vi "string test.vi"(11 "Array":string[][](array[string])) -> (2 "Modified Array Out":dbl[](array[numeric])=[2.0], 3 "Location":i32[][](array[numeric]))   [LabVIEW 2012]
uses:
  <vilib>/regexp/Match Regular Expression.xnode
panel:
  out "x >= 0?":bool
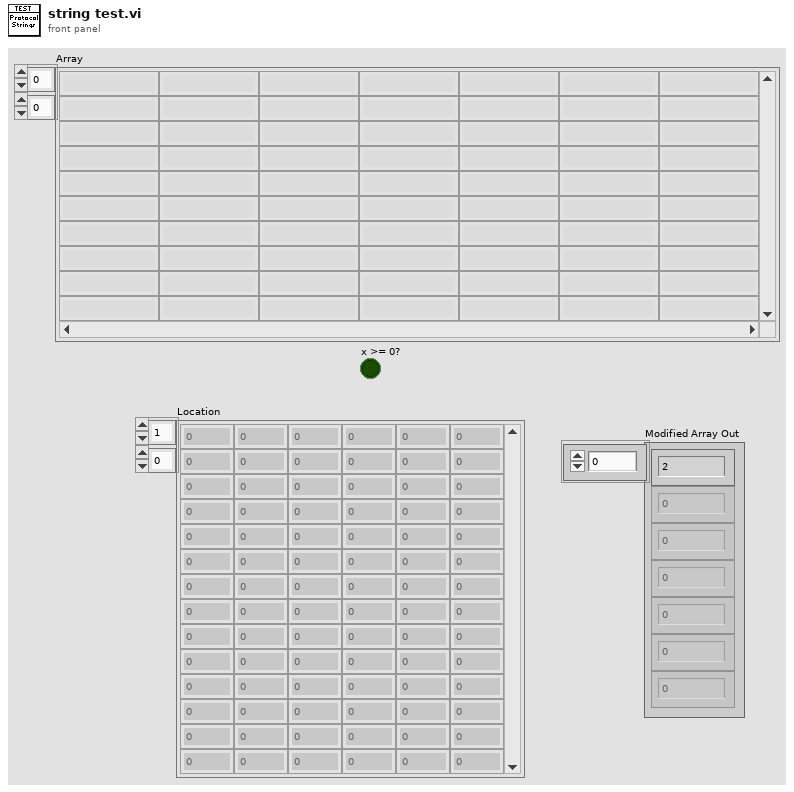
[diagram p1: front panel]
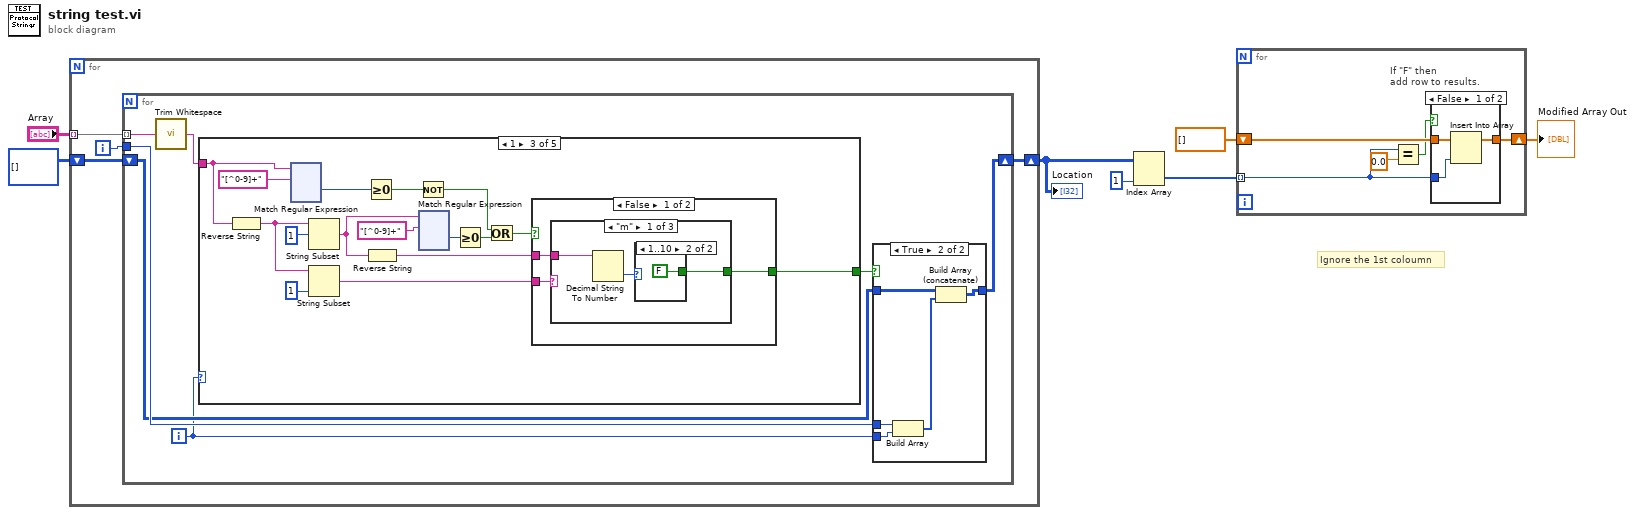
[diagram p0: block diagram]
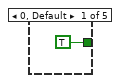
[diagram p4: hidden frame]
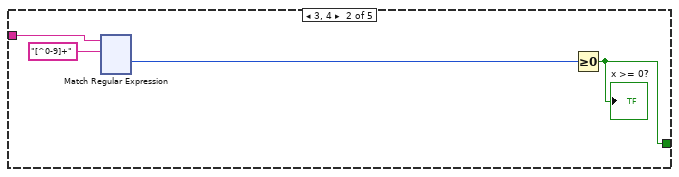
[diagram p5: hidden frame]
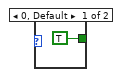
[diagram p6: hidden frame]
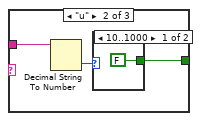
[diagram p7: hidden frame]
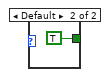
[diagram p8: hidden frame]
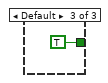
[diagram p9: hidden frame]
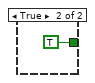
[diagram p10: hidden frame]
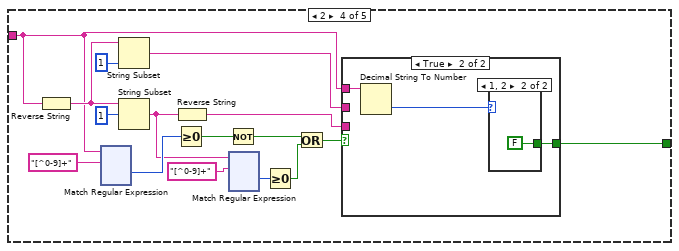
[diagram p11: hidden frame]
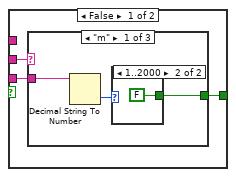
[diagram p12: hidden frame]
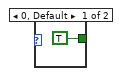
[diagram p13: hidden frame]
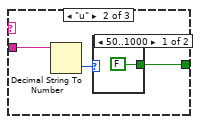
[diagram p14: hidden frame]
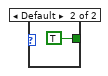
[diagram p15: hidden frame]
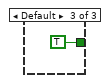
[diagram p16: hidden frame]
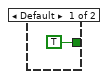
[diagram p17: hidden frame]
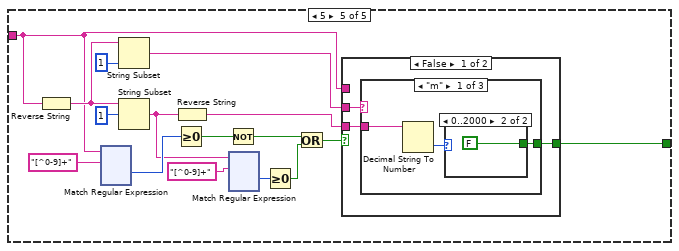
[diagram p18: hidden frame]
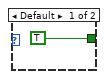
[diagram p19: hidden frame]
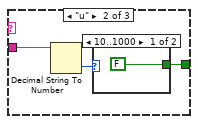
[diagram p20: hidden frame]
diagram:
  # "Ignore the 1st coloumn"
  n1 = for {
    tunnel: "Array" -> [w11] mode=indexing
    shift-right: [w8] -> w3
    shift-left: i32[][] [] -> [w9]
    i -> [w10]
    n2 = for {
      tunnel: w11 -> [w18] mode=indexing
      tunnel: w10 -> [w17]
      shift-right: [w16] -> w8
      shift-left: w9 -> [w15]
      i -> [w14]
      n3 = call <vilib>:"Trim Whitespace.vi"("string"=w18) -> ("trimmed string"=w13:string)  [unwired: 1 in]
      n4 = case shown="1" w14 {
        tunnel: w13 -> [_ w27 w151 w394 w651]
        tunnel: [TRUE ("y") w26 w152 w405 w662] -> w12
        frame 0, Default {
        }
        frame 3, 4 {
          n5 = xnode "Match Regular Expression"("input string"=w27, "regular expression"="[^0-9]+") -> ("offset past match"=w29:i32)  [unwired: 4 in, 4 out]
          n6 = Greater Or Equal To 0?(x=w29) -> (x >= 0?=w26:bool)
          "x >= 0?" <- w26
        }
        frame 1 {
          n7 = Reverse String(1:w151) -> (0:w149:string)
          n8 = xnode "Match Regular Expression"("input string"=w151, "regular expression"="[^0-9]+") -> ("offset past match"=w156:i32)  [unwired: 4 in, 4 out]
          n9 = String Subset(string=w149, offset (0)=1) -> (substring=w143:string)  [unwired: 1 in]
          n10 = String Subset(string=w149, length (rest)=1 ("length (rest)")) -> (substring=w153:string)  [unwired: 1 in]
          n11 = Greater Or Equal To 0?(x=w156) -> (x >= 0?=w150:bool)
          n12 = Reverse String(1:w143) -> (0:w142:string)
          n13 = Not(x=w150) -> (.not. x?=w144:bool)
          n14 = xnode "Match Regular Expression"("input string"=w143, "regular expression"="[^0-9]+") -> ("offset past match"=w147:i32)  [unwired: 4 in, 4 out]
          n15 = Greater Or Equal To 0?(x=w147) -> (x >= 0?=w145:bool)
          n16 = Or(x=w144, y=w145) -> (x .or. y?=w141:bool)
          n17 = case shown="False" w141 {
            tunnel: w153 -> [w270 _]
            tunnel: [w269 TRUE ("y")] -> w152
            tunnel: w142 -> [w268 _]
            frame False {
              n18 = case shown="\"m\"" w270 {
                tunnel: [w272 w277 TRUE ("y")] -> w269
                tunnel: w268 -> [w271 w276 _]
                frame "m" {
                  n19 = Decimal String To Number(string=w271) -> (number=w273:i32)  [unwired: 2 in, 1 out]
                  n20 = case shown="1..10" w273 {
                    tunnel: [TRUE ("y") FALSE ("y")] -> w272
                    frame 0, Default {
                    }
                    frame 1..10 {
                    }
                  }
                }
                frame "u" {
                  n21 = Decimal String To Number(string=w276) -> (number=w278:i32)  [unwired: 2 in, 1 out]
                  n22 = case shown="10..1000" w278 {
                    tunnel: [FALSE ("y") TRUE ("y")] -> w277
                    frame 10..1000 {
                    }
                    frame Default {
                    }
                  }
                }
                frame Default {
                }
              }
            }
            frame True {
            }
          }
        }
        frame 2 {
          n23 = Reverse String(1:w394) -> (0:w403:string)
          n24 = xnode "Match Regular Expression"("input string"=w394, "regular expression"="[^0-9]+") -> ("offset past match"=w409:i32)  [unwired: 4 in, 4 out]
          n25 = String Subset(string=w403, length (rest)=1 ("length (rest)")) -> (substring=w406:string)  [unwired: 1 in]
          n26 = String Subset(string=w403, offset (0)=1) -> (substring=w397:string)  [unwired: 1 in]
          n27 = Greater Or Equal To 0?(x=w409) -> (x >= 0?=w404:bool)
          n28 = Reverse String(1:w397) -> (0:w396:string)
          n29 = Not(x=w404) -> (.not. x?=w398:bool)
          n30 = xnode "Match Regular Expression"("input string"=w397, "regular expression"="[^0-9]+") -> ("offset past match"=w401:i32)  [unwired: 4 in, 4 out]
          n31 = Greater Or Equal To 0?(x=w401) -> (x >= 0?=w399:bool)
          n32 = Or(x=w398, y=w399) -> (x .or. y?=w395:bool)
          n33 = case shown="True" w395 {
            tunnel: w406 -> [w523 _]
            tunnel: [w522 w537] -> w405
            tunnel: w396 -> [w521 _]
            tunnel: w394 -> [_ w536]
            frame False {
              n34 = case shown="\"m\"" w523 {
                tunnel: [w525 w530 TRUE ("y")] -> w522
                tunnel: w521 -> [w524 w529 _]
                frame "m" {
                  n35 = Decimal String To Number(string=w524) -> (number=w526:i32)  [unwired: 2 in, 1 out]
                  n36 = case shown="1..2000" w526 {
                    tunnel: [TRUE ("y") FALSE ("y")] -> w525
                    frame 0, Default {
                    }
                    frame 1..2000 {
                    }
                  }
                }
                frame "u" {
                  n37 = Decimal String To Number(string=w529) -> (number=w531:i32)  [unwired: 2 in, 1 out]
                  n38 = case shown="50..1000" w531 {
                    tunnel: [FALSE ("y") TRUE ("y")] -> w530
                    frame 50..1000 {
                    }
                    frame Default {
                    }
                  }
                }
                frame Default {
                }
              }
            }
            frame True {
              n39 = Decimal String To Number(string=w536) -> (number=w535:i32)  [unwired: 2 in, 1 out]
              n40 = case shown="1, 2" w535 {
                tunnel: [TRUE ("y") FALSE ("y")] -> w537
                frame Default {
                }
                frame 1, 2 {
                }
              }
            }
          }
        }
        frame 5 {
          n41 = Reverse String(1:w651) -> (0:w660:string)
          n42 = xnode "Match Regular Expression"("input string"=w651, "regular expression"="[^0-9]+") -> ("offset past match"=w666:i32)  [unwired: 4 in, 4 out]
          n43 = String Subset(string=w660, length (rest)=1 ("length (rest)")) -> (substring=w663:string)  [unwired: 1 in]
          n44 = String Subset(string=w660, offset (0)=1) -> (substring=w654:string)  [unwired: 1 in]
          n45 = Greater Or Equal To 0?(x=w666) -> (x >= 0?=w661:bool)
          n46 = Reverse String(1:w654) -> (0:w653:string)
          n47 = Not(x=w661) -> (.not. x?=w655:bool)
          n48 = xnode "Match Regular Expression"("input string"=w654, "regular expression"="[^0-9]+") -> ("offset past match"=w658:i32)  [unwired: 4 in, 4 out]
          n49 = Greater Or Equal To 0?(x=w658) -> (x >= 0?=w656:bool)
          n50 = Or(x=w655, y=w656) -> (x .or. y?=w652:bool)
          n51 = case shown="False" w652 {
            tunnel: w663 -> [w780 _]
            tunnel: [w779 w794] -> w662
            tunnel: w653 -> [w778 _]
            tunnel: w651 -> [_ w793]
            frame False {
              n52 = case shown="\"m\"" w780 {
                tunnel: [w782 w787 TRUE ("y")] -> w779
                tunnel: w778 -> [w781 w786 _]
                frame "m" {
                  n53 = Decimal String To Number(string=w781) -> (number=w783:i32)  [unwired: 2 in, 1 out]
                  n54 = case shown="0..2000" w783 {
                    tunnel: [TRUE ("y") FALSE ("y")] -> w782
                    frame Default {
                    }
                    frame 0..2000 {
                    }
                  }
                }
                frame "u" {
                  n55 = Decimal String To Number(string=w786) -> (number=w788:i32)  [unwired: 2 in, 1 out]
                  n56 = case shown="10..1000" w788 {
                    tunnel: [FALSE ("y") TRUE ("y")] -> w787
                    frame 10..1000 {
                    }
                    frame Default {
                    }
                  }
                }
                frame Default {
                }
              }
            }
            frame True {
              n57 = Decimal String To Number(string=w793) -> (number=w792:i32)  [unwired: 2 in, 1 out]
              n58 = case shown="1" w792 {
                tunnel: [TRUE ("y") FALSE ("y")] -> w794
                frame Default {
                }
                frame 1 {
                }
              }
            }
          }
        }
      }
      n59 = case shown="True" w12 {
        tunnel: w14 -> [_ w23]
        tunnel: w17 -> [_ w24]
        tunnel: [w19 w22] -> w16
        tunnel: w15 -> [w19 w21]
        frame False {
        }
        frame True {
          n60 = Build Array(w24, w23) -> (w20:i32[])
          n61 = Build Array (concatenate)(w21, w20) -> (w22:i32[][])
        }
      }
    }
  }
  "Location" <- w3
  n62 = Index Array(array=w3, index (col)=1 ("disabled index (col)")) -> (element=w1:i32[])  [unwired: 1 in]
  n63 = for {
    tunnel: w1 -> [w910] mode=indexing
    shift-right: [w911] -> w4
    shift-left: dbl[] [] ("Storage Array") -> [w912]
    n64 = Equal?(x=w910, y=0.0) -> (x = y?=w908:bool)
    n65 = case "If \"F\" then \nadd row to results." shown="False" w908 {
      tunnel: w912 -> [w915 w916]
      tunnel: w910 -> [w914 _]
      tunnel: [w913 w916] -> w911
      frame False {
        n66 = Insert Into Array(array=w915, new element=w914) -> (w913:dbl[])  [unwired: 1 in]
      }
      frame True {
      }
    }
  }
  "Modified Array Out" <- w4
